vi "ReadFromLockin.vi"(4 "#Measurements each Frequency":i32=200, 5 "Path":path, 7 "Frequency":dbl=200.0 format="%.2f", 8 "error in 2":errorcluster) -> (0 "error out 2":errorcluster)   [LabVIEW 2010]
uses:
  <vilib>/Utility/file.llb/Write To Spreadsheet File (DBL).vi
  <vilib>/Analysis/NI_AALBase.lvlib
panel:
  out "Phase phi":dbl=200.0 format="%.2f"
  out "Amplitude A":dbl=200.0 format="%.2f"
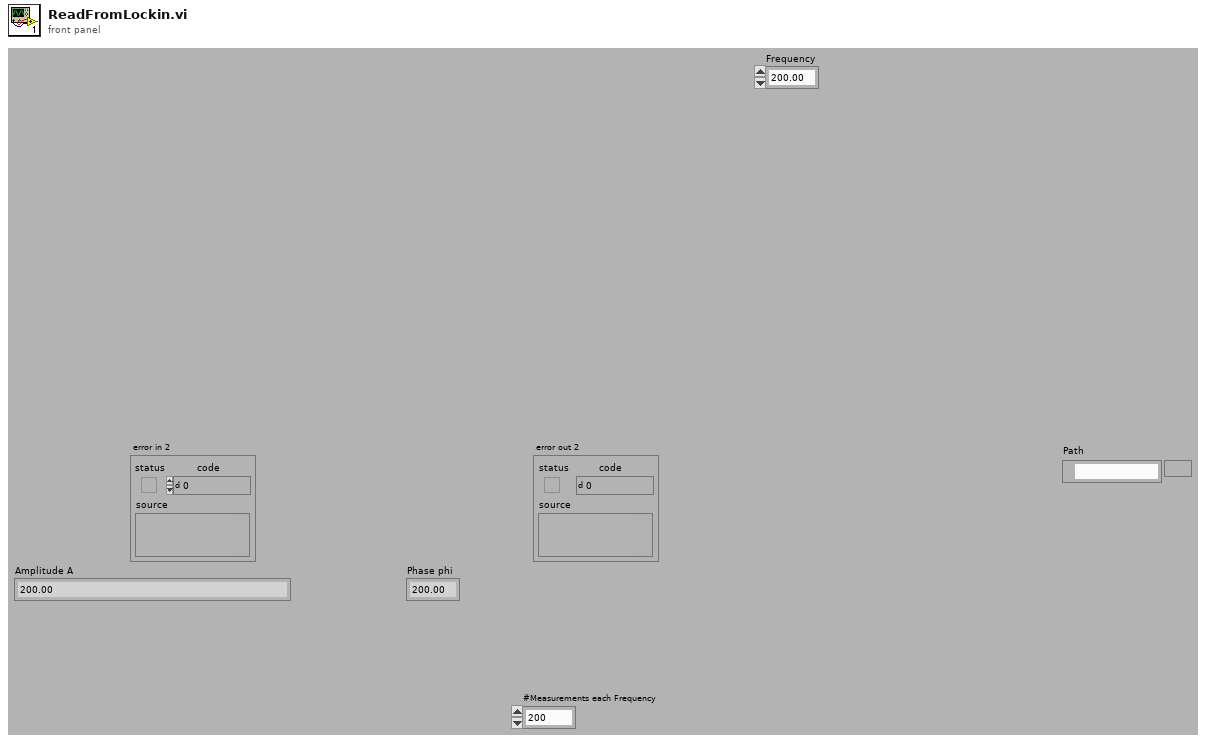
[diagram p1: front panel]
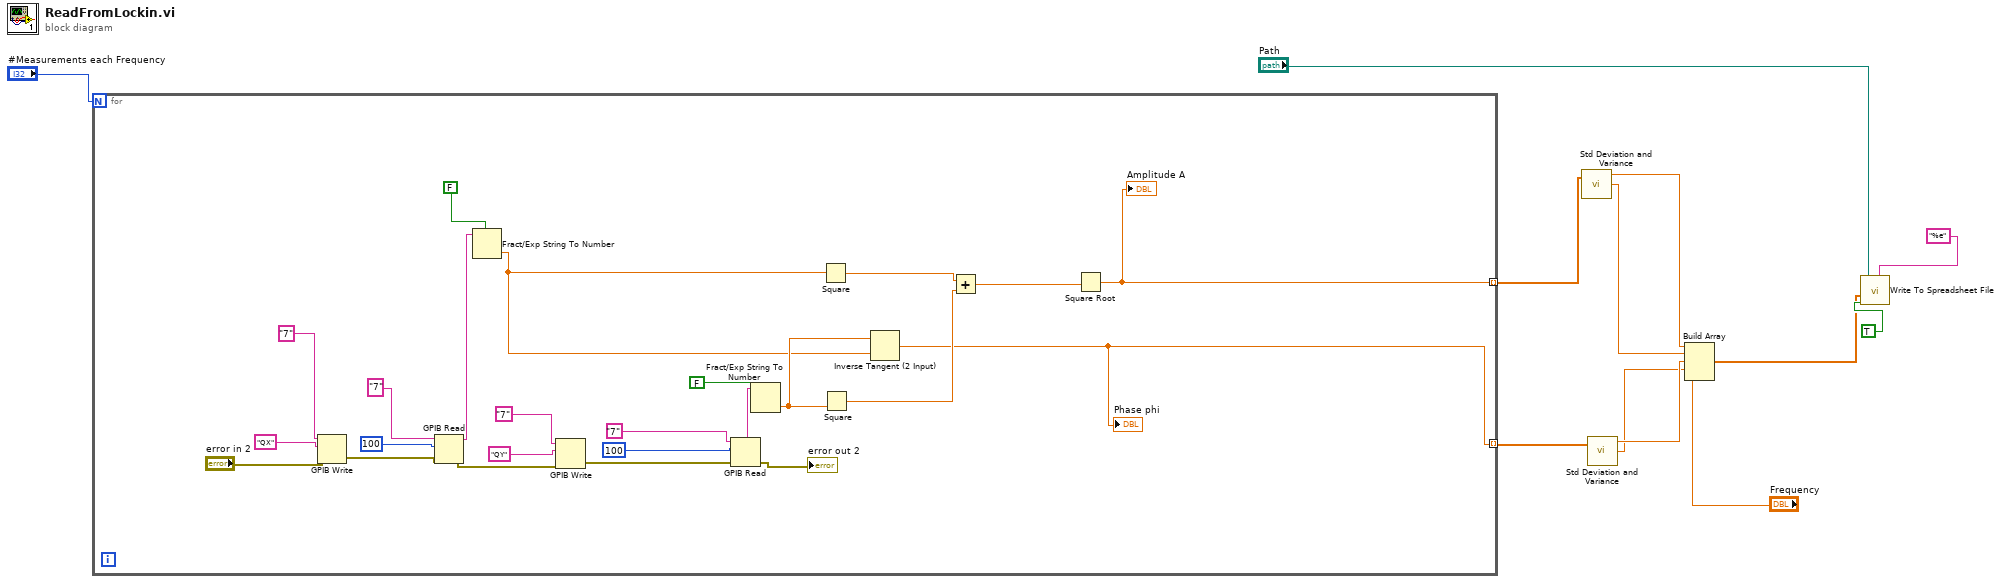
[diagram p0: block diagram]
diagram:
  n1 = for {
    N: "#Measurements each Frequency" -> [_]
    tunnel: [w14] -> w8 mode=indexing
    tunnel: [w13] -> w7 mode=indexing
    n2 = GPIB Write(0:"7", 1:"QX", 3:"error in 2") -> (6:w35:errorcluster)  [unwired: 2 in, 1 out]
    n3 = GPIB Read(0:"7", 1:100, 3:w35) -> (5:w33:string, 7:w34:errorcluster)  [unwired: 2 in, 1 out]
    n4 = Fract/Exp String To Number(use system decimal point (T)=FALSE, string=w33) -> (number=w16:dbl)  [unwired: 2 in, 1 out]
    n5 = GPIB Write(0:"7", 1:"QY", 3:w34) -> (6:w22:errorcluster)  [unwired: 2 in, 1 out]
    n6 = GPIB Read(0:"7", 1:100, 3:w22) -> (5:w19:string, 7:→"error out 2":errorcluster)  [unwired: 2 in, 1 out]
    n7 = Fract/Exp String To Number(use system decimal point (T)=FALSE, string=w19) -> (number=w30:dbl)  [unwired: 2 in, 1 out]
    n8 = Square(x=w16) -> (x^2=w15:dbl)
    n9 = Square(x=w30) -> (x^2=w29:dbl)
    n10 = Inverse Tangent (2 Input)(1:w16, 2:w30) -> (0:w13:dbl)
    "Phase phi" <- w13
    n11 = Add(x=w15, y=w29) -> (x+y=w17:dbl)
    n12 = Square Root(x=w17) -> (sqrt(x)=w14:dbl)
    "Amplitude A" <- w14
  }
  n13 = call <vilib>:"Std Deviation and Variance.vi"("X"=w8) -> ("mean"=w6:dbl, "standard deviation"=w5:dbl)  [unwired: 1 in, 1 out]
  n14 = call <vilib>:"Std Deviation and Variance.vi"("X"=w7) -> ("mean"=w3:dbl, "standard deviation"=w2:dbl)  [unwired: 1 in, 1 out]
  n15 = Build Array(w6, w5, w3, w2, "Frequency") -> (w4:dbl[])
  n16 = call-poly <vilib>:"Write To Spreadsheet File.vi"("format (%.3f)"="%e", "append to file? (new file:F)"=TRUE, "1D data"=w4, "file path (dialog if empty)"="Path") -> ()  [unwired: 4 in, 1 out]
